vi "Puff_release3_chs.vi"() -> (5 "Plug in titles":string[](array[string]), 7 "Plug in values":string[](array[string]))   [LabVIEW 2011]
uses:
  Controls/Post_Process.ctl
  Globals/Plug_in_data_global.vi
  Globals/Meas_global.vi
  Globals/Constants_global.vi
  Globals/Dynamic_call_global.ph.vi
  <vilib>/Analysis/NI_AALPro.lvlib
panel:
  out "FFID Trace Variance":cluster{dbl, dbl, dbl[]}(graph)
  in  "Per Block Mode":T1(ring)
  in  "Averaging Samples":i32=1 min=1
  out "Valve to monitor delay (s)":dbl format="%.2f"
  out "Monitor trigger Index":dbl format="%.2f"
  out "Valve Trigger Index":dbl format="%.2f"
  out "Monitor FID":cluster{dbl, dbl, dbl[]}(graph)
  out "delay":dbl format="%.2f"
  out "Pulse Width":dbl format="%.2f"
  out "falltime":dbl format="%.2f"
  out "top":dbl format="%.2f"
  out "risetime":dbl format="%.2f"
  in  "Save Time pdf?":bool
  out "Pdf":cluster{"Axis":dbl[], dbl[]}(graph)
  in  "Histogram Time":dbl format="%.2f"
  out "Current Block No":i32
  in  "Save averaged traces?":bool
  in  "Pause Mode":T2(ring)
  in  "OK":bool
  out "No of Valid Blocks":dbl
  out "Valve Trace":dbl[](graph)
  out "FFID Trace":cluster{dbl, dbl, dbl[]}(graph)
  out "Source On":i32
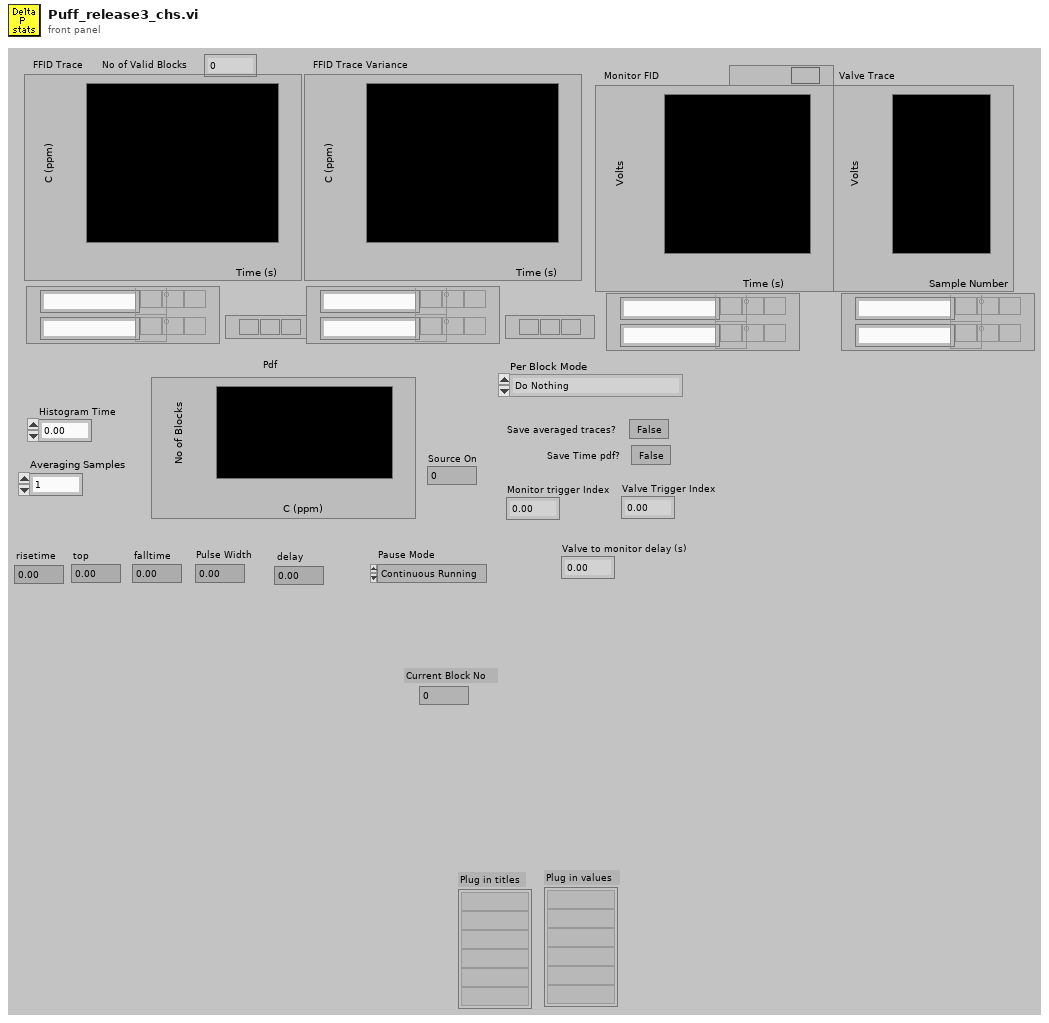
[diagram p1: front panel]
types:
  T1 = enum16{"Do Nothing", "Save Block Time Traces", "Save Jpeg plots"}
  T2 = enum16{"Continuous Running", "After Each  Block"}
  T3 = typedef "Post_Process.ctl" = enum16{"Take New Data", "Post Process Raw Data File"}
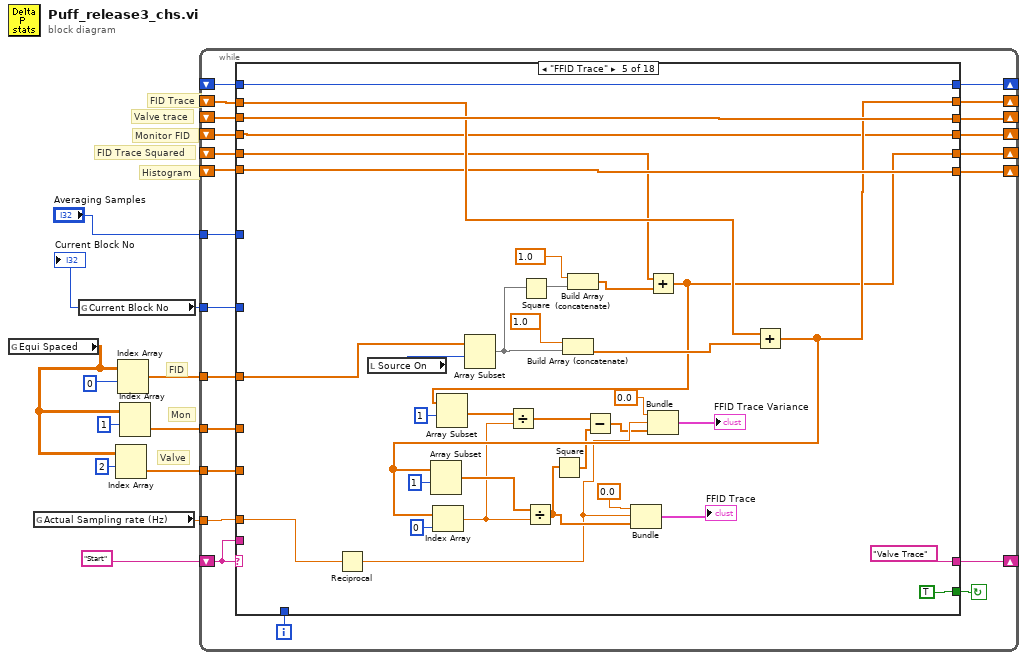
[diagram p0: block diagram]
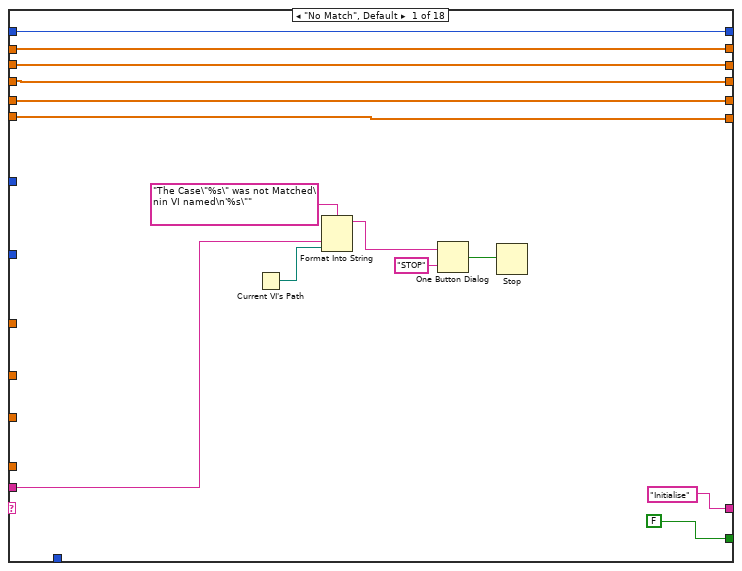
[diagram p2: hidden frame]
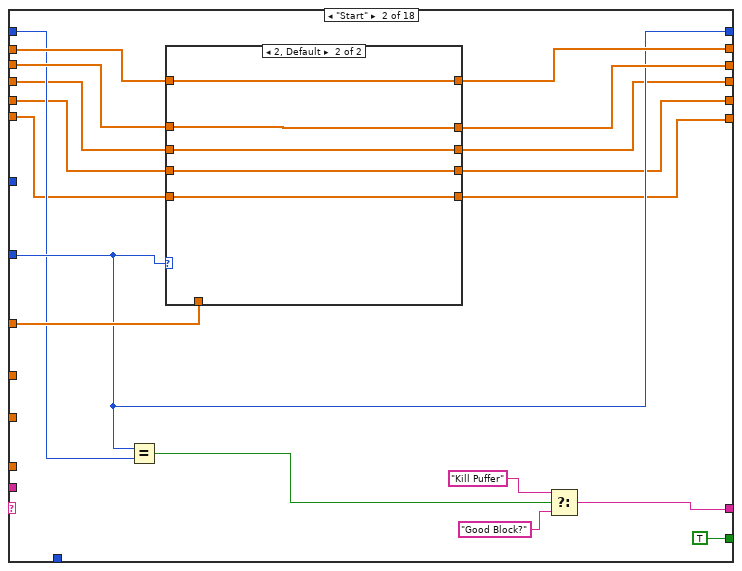
[diagram p3: hidden frame]
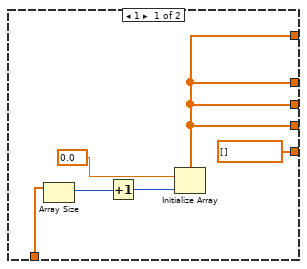
[diagram p4: hidden frame]
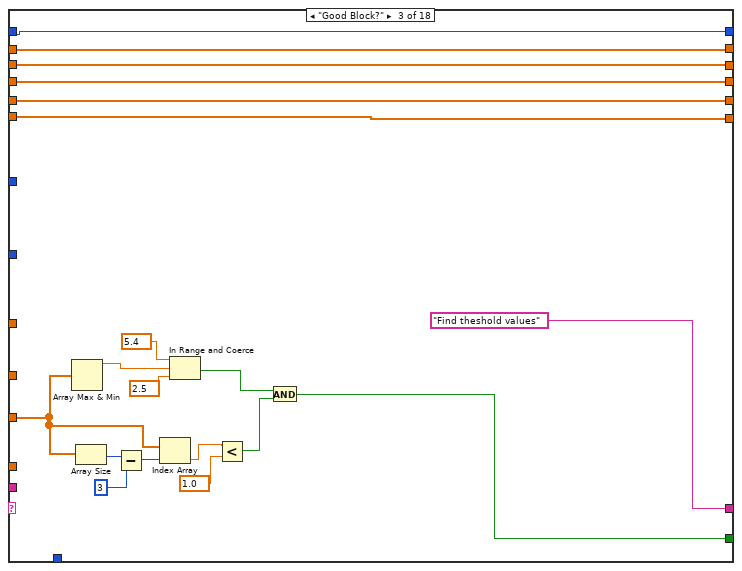
[diagram p5: hidden frame]
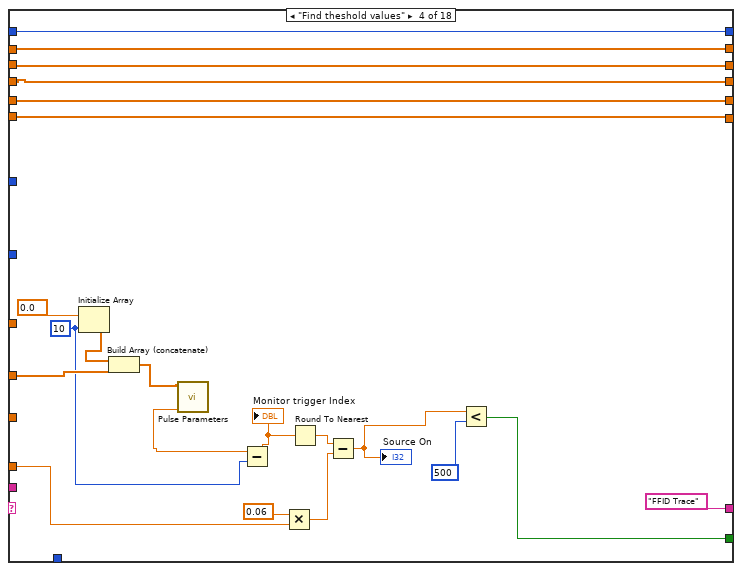
[diagram p6: hidden frame]
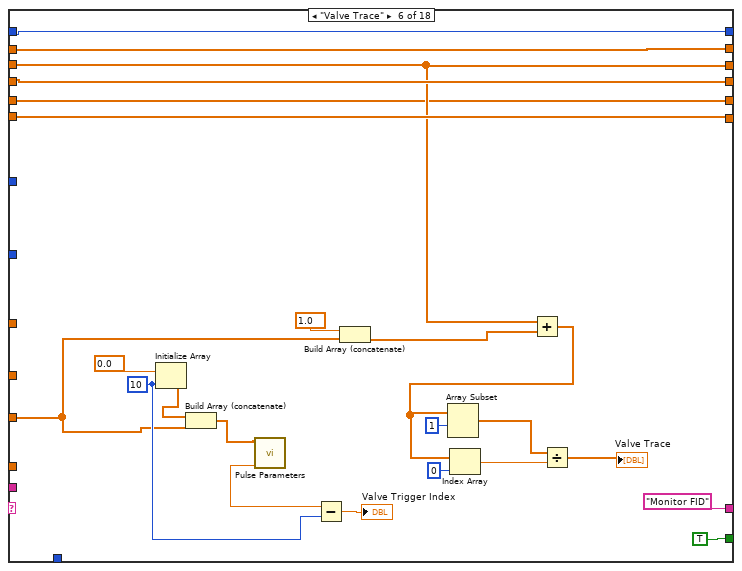
[diagram p7: hidden frame]
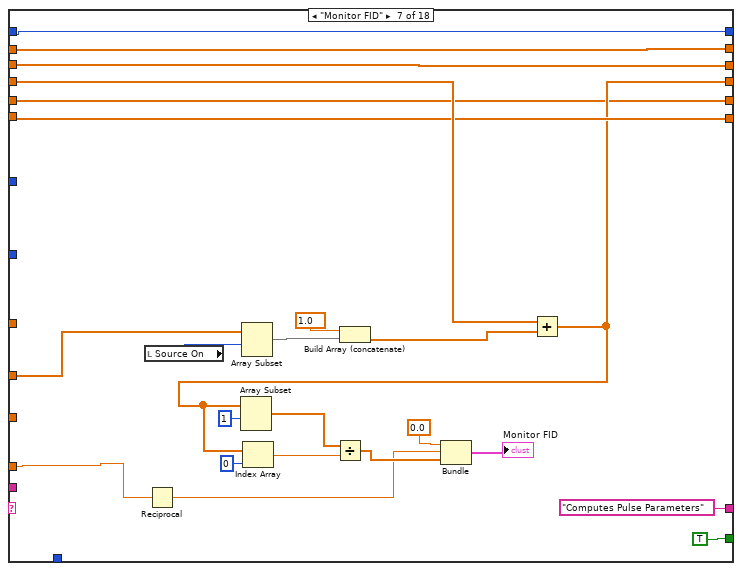
[diagram p8: hidden frame]
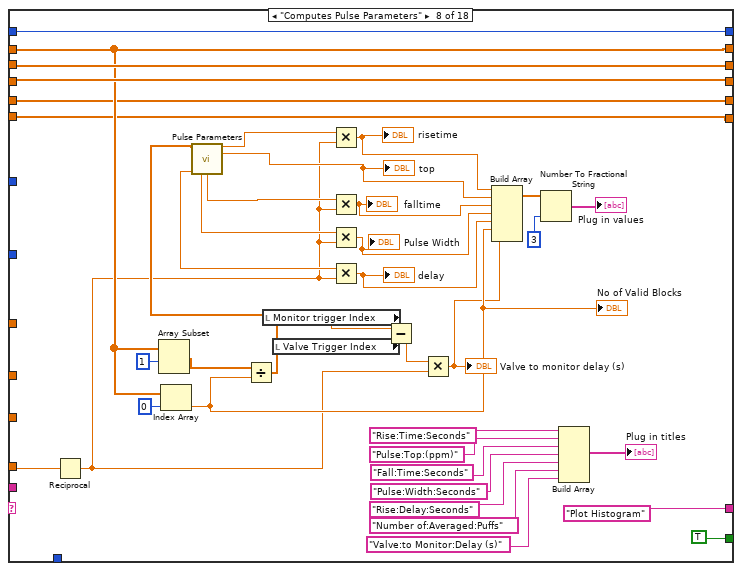
[diagram p9: hidden frame]
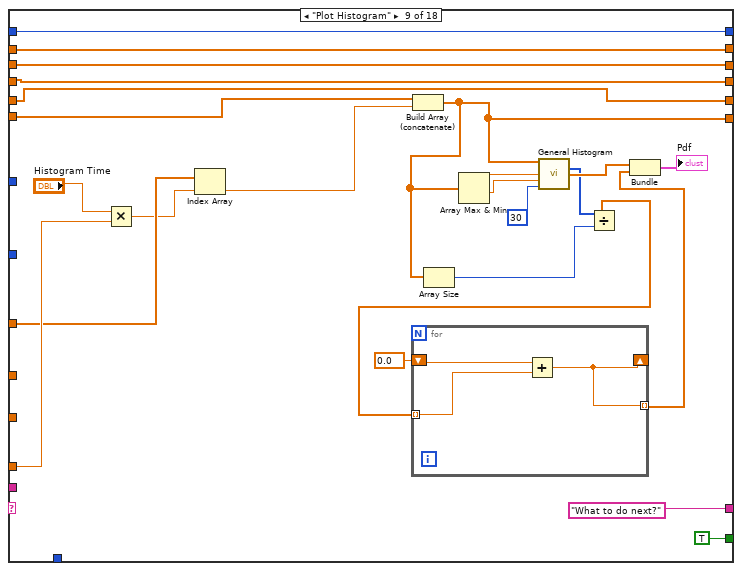
[diagram p10: hidden frame]
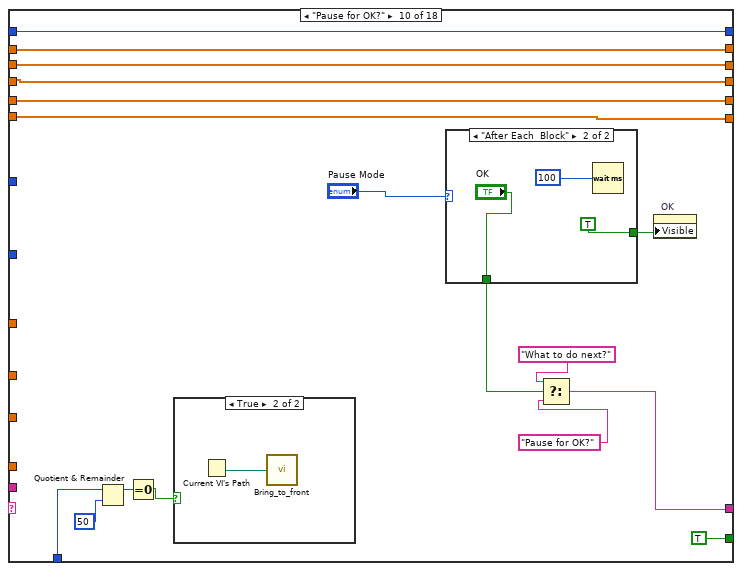
[diagram p11: hidden frame]
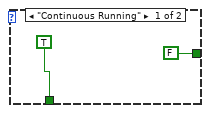
[diagram p13: hidden frame]
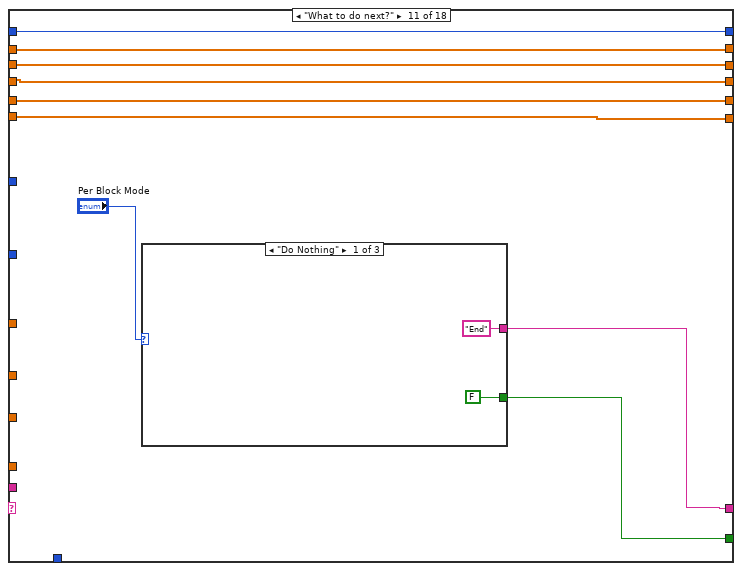
[diagram p14: hidden frame]
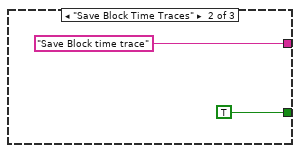
[diagram p15: hidden frame]
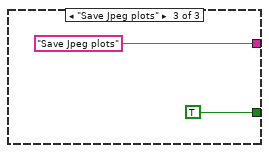
[diagram p16: hidden frame]
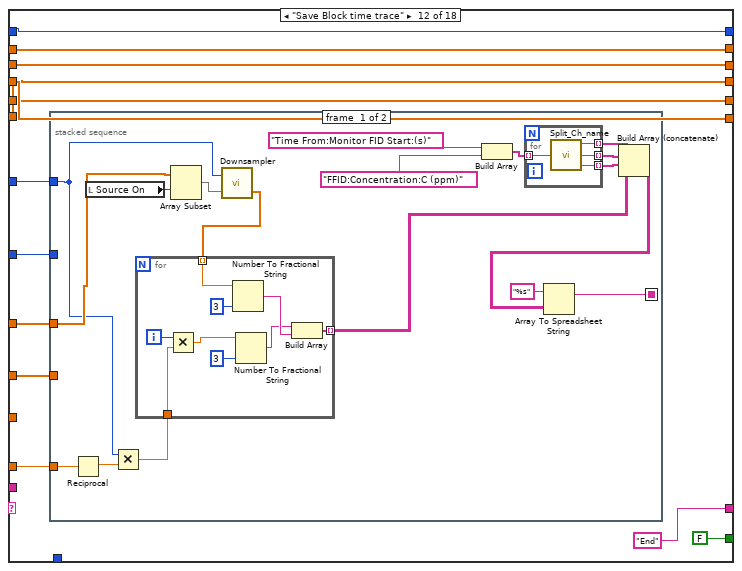
[diagram p17: hidden frame]
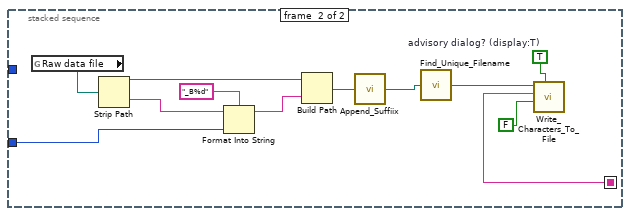
[diagram p18: hidden frame]
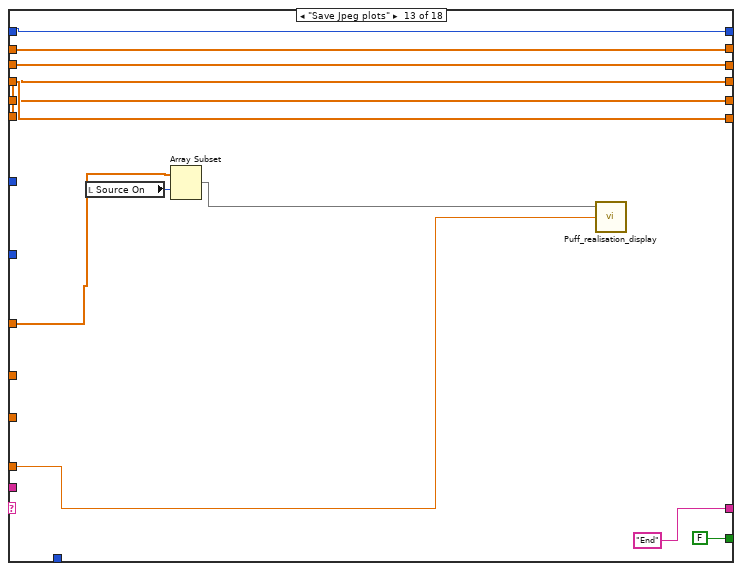
[diagram p19: hidden frame]
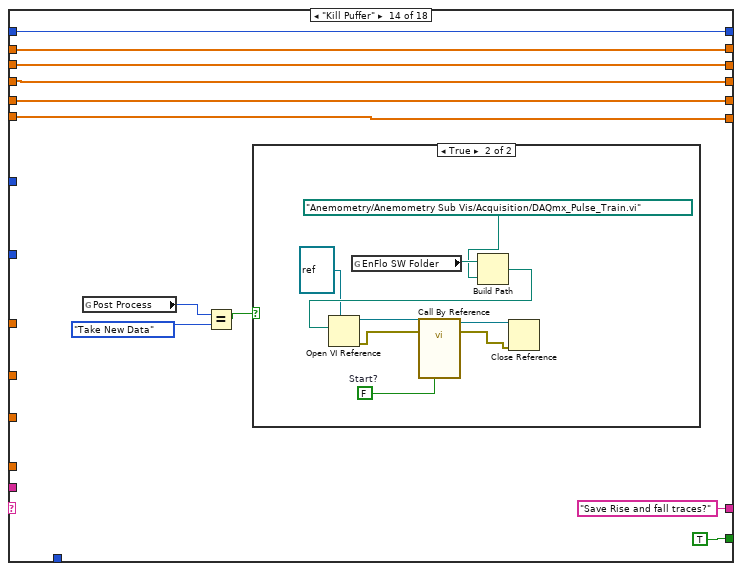
[diagram p20: hidden frame]
diagram:
  # "FID Trace Squared"
  # "Valve"
  # "Mon"
  # "FID"
  # "Histogram"
  # "Monitor FID"
  # "Valve trace"
  # "FID Trace"
  n1 = global read "Plug_in_data_global.vi" "Equi Spaced"() -> (w4:dbl[][])
  n2 = global read "Meas_global.vi" "Actual Sampling rate (Hz)"() -> (w8:dbl)
  n3 = global read "Meas_global.vi" "Current Block No"() -> (w7:i32)
  "Current Block No" <- w7
  n4 = Index Array(array=w4, index (row)=2) -> (element=w3:dbl[])  [unwired: 1 in]
  n5 = Index Array(array=w4, index (row)=0) -> (element=w9:dbl[])  [unwired: 1 in]
  n6 = Index Array(array=w4, index (row)=1) -> (element=w10:dbl[])  [unwired: 1 in]
  n7 = while {
    shift-left: "Start" -> [w31]
    shift-right: [w32] -> _
    shift-right: [w30] -> _
    shift-left: _ -> [w27]
    shift-right: [w29] -> _
    shift-left: _ -> [w28]
    tunnel: w10 -> [w26]
    tunnel: w9 -> [w25]
    tunnel: w8 -> [w24]
    tunnel: w7 -> [w23]
    shift-right: [w20] -> _
    shift-left: _ -> [w21]
    shift-right: [w18] -> _
    shift-left: _ -> [w19]
    shift-right: [w16] -> _
    shift-left: _ -> [w15]
    tunnel: w3 -> [w17]
    tunnel: "Averaging Samples" -> [w14]
    shift-right: [w12] -> _
    shift-left: _ -> [w13]
    i -> [w22]
    stop <- w33 continue-if-true
    n8 = case shown="\"FFID Trace\"" w31 {
      tunnel: [FALSE TRUE ("Processing last block?") w85 w112 TRUE ("Processing last block?") TRUE ("Processing last block?") TRUE ("Processing last block?") TRUE ("Processing last block?") TRUE ("Processing last block?") TRUE ("Processing last block?") w287 FALSE ("Processing last block?") FALSE ("Processing last block?") TRUE ("Processing last block?") w390 TRUE ("Processing last block?") "Save Time pdf?" FALSE ("Processing last block?")] -> w33
      tunnel: ["Initialise" w55 "Find theshold values" "FFID Trace" "Valve Trace" "Monitor FID" "Computes Pulse Parameters" "Plot Histogram" ("f") "What to do next?" ("f") w266 w288 "End" "End" "Save Rise and fall traces?" w393 "Save Time pdf?" "Save Time pdf" "End"] -> w32
      tunnel: w31 -> [w42 _ _ _ _ _ _ _ _ _ _ _ _ _ _ _ _ _]
      tunnel: [w39 w64 w95 w115 w137 w170 w191 w205 w259 w279 w294 w313 w368 w379 w399 w407 w477 w488] -> w30
      tunnel: [w38 w62 w94 w114 w148 w152 w188 w233 w258 w278 w293 w312 w367 w378 w398 w406 w476 w487] -> w29
      tunnel: w28 -> [w38 w61 w94 w114 w148 w152 w188 w233 w258 w278 w293 w312 w367 w378 w398 w406 w476 w487]
      tunnel: w27 -> [w39 w63 w95 w115 w146 w170 w191 w205 w259 w279 w294 w313 w368 w379 w399 w407 w477 w488]
      tunnel: w26 -> [_ _ _ w108 _ _ w175 _ _ _ _ w309 _ _ _ _ _ w484]
      tunnel: w25 -> [_ w60 _ _ w147 _ _ _ w254 _ _ w308 w361 _ _ _ _ w483]
      tunnel: w24 -> [_ _ _ w102 w135 _ w176 w231 w255 _ _ w302 w358 _ _ _ _ _]
      tunnel: w23 -> [_ w59 _ _ _ _ _ _ _ _ _ w307 _ _ _ _ _ w482]
      tunnel: w22 -> [_ _ _ _ _ _ _ _ _ w276 _ _ _ _ _ _ _ _]
      tunnel: w21 -> [w37 w58 w86 w111 w142 w169 w190 w229 w257 w272 w292 w306 w364 w375 _ w403 _ w481]
      tunnel: [w37 w59 w86 w111 w142 w169 w190 w229 w257 w272 w292 w306 w364 w375 0 w403 0 w481] -> w20
      tunnel: w19 -> [w36 w52 w84 w104 w141 w162 w186 w204 w251 w271 w291 w305 w363 w371 w391 w402 w472 w479]
      tunnel: [w36 w53 w84 w104 w141 w162 w186 w204 w243 w271 w291 w305 w363 w371 w391 w402 w472 w479] -> w18
      tunnel: w17 -> [_ _ w80 _ _ w155 _ _ _ _ _ _ _ _ _ _ _ _]
      tunnel: [w35 w51 w81 w105 w133 w163 w177 w209 w240 w270 w290 w304 w362 w370 w392 w401 w471 w480] -> w16
      tunnel: w15 -> [w35 w50 w81 w105 w133 w163 w187 w209 w240 w270 w290 w304 w362 w370 w392 w401 w471 w480]
      tunnel: w14 -> [_ _ _ _ _ _ _ _ _ _ _ w303 _ _ _ _ _ _]
      tunnel: w13 -> [w34 w48 w77 w96 w128 w151 w174 w197 w236 w263 w286 w301 w357 w369 w389 w400 w470 w478]
      tunnel: [w34 w49 w77 w96 w126 w151 w174 w197 w236 w263 w286 w301 w357 w369 w389 w400 w470 w478] -> w12
      frame "No Match", Default {
        n9 = Current VI's Path() -> (path=w41:path)
        n10 = Format Into String(format string="The Case\"%s\" was not Matched\nin VI named\n'%s\"" ("Format String"), w42, w41) -> (resulting string=w45:string)  [unwired: 2 in, 1 out]
        n11 = One Button Dialog(message=w45, button name ("OK")="STOP") -> (true=w43:bool)
        n12 = Stop(stop? (T)=w43) -> ()
      }
      frame "Start" {
        n13 = Equal?(x=w59, y=w58) -> (x = y?=w57:bool)
        n14 = case shown="2, Default" w59 {
          tunnel: [w66 w76] -> w64
          tunnel: w63 -> [_ w76]
          tunnel: [w66 w75] -> w62
          tunnel: w61 -> [_ w75]
          tunnel: w60 -> [w71 _]
          tunnel: [dbl[] [] w74] -> w53
          tunnel: w52 -> [_ w74]
          tunnel: [w66 w73] -> w51
          tunnel: w50 -> [_ w73]
          tunnel: [w66 w72] -> w49
          tunnel: w48 -> [_ w72]
          frame 1 {
            n15 = Array Size(array=w71) -> (size(s)=w70:i32)
            n16 = Increment(x=w70) -> (x+1=w67:i32)
            n17 = Initialize Array(0.0 ("element"), w67) -> (w66:dbl[])
          }
          frame 2, Default {
          }
        }
        n18 = Select(t="Kill Puffer", s=w57, f="Good Block?") -> (s? t:f=w55:string)
      }
      frame "Good Block?" {
        n19 = Array Max & Min(array=w80) -> (max value=w83:dbl)  [unwired: 3 out]
        n20 = Array Size(array=w80) -> (size(s)=w79:i32)
        n21 = Subtract(x=w79, y=3) -> (x-y=w91:i32)
        n22 = Index Array(array=w80, index=w91) -> (element=w90:dbl)
        n23 = In Range and Coerce(upper limit=5.4, x=w83, lower limit=2.5 ("y")) -> (In Range?=w87:bool)  [unwired: 1 out]
        n24 = Less?(x=w90, y=1.0) -> (x < y?=w88:bool)
        n25 = And(x=w87, y=w88) -> (x .and. y?=w85:bool)
      }
      frame "Find theshold values" {
        w106 = 10 ("dimension size")
        n26 = Initialize Array(0.0, w106) -> (w107:dbl[])
        n27 = Build Array (concatenate)(w107, w108) -> (w109:dbl[])
        n28 = call <vilib>:"Pulse Parameters.vi"("X"=w109) -> ("delay"=w101:dbl)  [unwired: 14 out]
        n29 = Subtract(x=w101, y=w106) -> (x-y=w100:dbl)
        "Monitor trigger Index" <- w100
        n30 = Multiply(x=0.06 ("y"), y=w102) -> (x*y=w98:dbl)
        n31 = Round To Nearest(number=w100) -> (nearest integer value=w99:dbl)
        n32 = Subtract(x=w99, y=w98) -> (x-y=w97:dbl)
        "Source On" <- w97
        n33 = Less?(x=w97, y=500) -> (x < y?=w112:bool)
      }
      frame "FFID Trace" {
        n34 = Reciprocal(x=w135) -> (1/x=w119:dbl)
        n35 = local read "Source On"() -> (w143:i32)
        n36 = Array Subset(array=w147, index=w143) -> (w131:dbl[])  [unwired: 1 in]
        n37 = Square(x=w131) -> (x^2=w130:dbl[])
        n38 = Build Array (concatenate)(1.0, w131) -> (w144:dbl[])
        n39 = Build Array (concatenate)(1.0, w130) -> (w129:dbl[])
        n40 = Add(x=w128, y=w129) -> (x+y=w126:dbl[])
        n41 = Array Subset(array=w126, index=1) -> (w125:dbl[])  [unwired: 1 in]
        n42 = Add(x=w146, y=w144) -> (x+y=w137:dbl[])
        n43 = Array Subset(array=w137, index=1) -> (w136:dbl[])  [unwired: 1 in]
        n44 = Index Array(array=w137, index=0) -> (element=w124:dbl)
        n45 = Divide(x=w125, y=w124) -> (x/y=w122:dbl[])
        n46 = Divide(x=w136, y=w124) -> (x/y=w123:dbl[])
        n47 = Square(x=w123) -> (x^2=w121:dbl[])
        n48 = Subtract(x=w122, y=w121) -> (x-y=w118:dbl[])
        n49 = Bundle(0.0, w119, w123) -> (→"FFID Trace":cluster{dbl, dbl, dbl[]})  [unwired: 1 out]
        n50 = Bundle(0.0, w119, w118) -> (→"FFID Trace Variance":cluster{dbl, dbl, dbl[]})  [unwired: 1 out]
      }
      frame "Valve Trace" {
        w156 = 10 ("dimension size")
        n51 = Initialize Array(0.0, w156) -> (w157:dbl[])
        n52 = Build Array (concatenate)(w157, w155) -> (w158:dbl[])
        n53 = call <vilib>:"Pulse Parameters.vi"("X"=w158) -> ("delay"=w153:dbl)  [unwired: 14 out]
        n54 = Subtract(x=w153, y=w156) -> (x-y=→"Valve Trigger Index":dbl)
        n55 = Build Array (concatenate)(1.0, w155) -> (w171:dbl[])
        n56 = Add(x=w152, y=w171) -> (x+y=w160:dbl[])
        n57 = Array Subset(array=w160, index=1) -> (w165:dbl[])  [unwired: 1 in]
        n58 = Index Array(array=w160, index=0) -> (element=w164:dbl)
        n59 = Divide(x=w165, y=w164) -> (x/y=→"Valve Trace":dbl[])
      }
      frame "Monitor FID" {
        n60 = local read "Source On"() -> (w193:i32)
        n61 = Reciprocal(x=w176) -> (1/x=w179:dbl)
        n62 = Array Subset(array=w175, index=w193) -> (w192:dbl[])  [unwired: 1 in]
        n63 = Build Array (concatenate)(1.0, w192) -> (w194:dbl[])
        n64 = Add(x=w187, y=w194) -> (x+y=w177:dbl[])
        n65 = Array Subset(array=w177, index=1) -> (w181:dbl[])  [unwired: 1 in]
        n66 = Index Array(array=w177, index=0) -> (element=w180:dbl)
        n67 = Divide(x=w181, y=w180) -> (x/y=w185:dbl[])
        n68 = Bundle(0.0, w179, w185) -> (→"Monitor FID":cluster{dbl, dbl, dbl[]})  [unwired: 1 out]
      }
      frame "Computes Pulse Parameters" {
        n69 = Reciprocal(x=w231) -> (1/x=w200:dbl)
        n70 = Array Subset(array=w205, index=1) -> (w208:dbl[])  [unwired: 1 in]
        n71 = Index Array(array=w205, index=0) -> (element=w207:dbl)
        "No of Valid Blocks" <- w207
        n72 = Divide(x=w208, y=w207) -> (x/y=w206:dbl[])
        n73 = call <vilib>:"Pulse Parameters.vi"("X"=w206) -> ("risetime"=w228:dbl, "top"=w214:dbl, "delay"=w225:dbl, "duration"=w226:dbl, "falltime"=w227:dbl)  [unwired: 10 out]
        "top" <- w214
        n74 = local read "Monitor trigger Index"() -> (w202:dbl)
        n75 = local read "Valve Trigger Index"() -> (w203:dbl)
        n76 = Multiply(x=w228, y=w200) -> (x*y=w213:dbl)
        "risetime" <- w213
        n77 = Multiply(x=w227, y=w200) -> (x*y=w212:dbl)
        "falltime" <- w212
        n78 = Multiply(x=w226, y=w200) -> (x*y=w211:dbl)
        "Pulse Width" <- w211
        n79 = Multiply(x=w225, y=w200) -> (x*y=w210:dbl)
        "delay" <- w210
        n80 = Subtract(x=w202, y=w203) -> (x-y=w201:dbl)
        n81 = Multiply(x=w201, y=w200) -> (x*y=w199:dbl)
        "Valve to monitor delay (s)" <- w199
        n82 = Build Array(w213, w214, w212, w211, w210, w207, w199) -> (w224:dbl[])
        n83 = Number To Fractional String(number=w224, precision (6)=i16 3) -> (F-format string=→"Plug in values":string[])  [unwired: 2 out]
        n84 = Build Array("Rise:Time:Seconds", "Pulse:Top:(ppm)", "Fall:Time:Seconds", "Pulse:Width:Seconds", "Rise:Delay:Seconds", "Number of:Averaged:Puffs", "Valve:to Monitor:Delay (s)") -> (→"Plug in titles":string[])
      }
      frame "Plot Histogram" {
        n85 = Multiply(x="Histogram Time", y=w255) -> (x*y=w253:dbl)
        n86 = Index Array(array=w254, index=w253) -> (element=w252:dbl)
        n87 = Build Array (concatenate)(w251, w252) -> (w243:dbl[])
        n88 = Array Size(array=w243) -> (size(s)=w241:i32)
        n89 = Array Max & Min(array=w243) -> (max value=w250:dbl, min value=w249:dbl)  [unwired: 2 out]
        n90 = call <vilib>:"General Histogram.vi"("X"=w243, "max"=w250, "min"=w249, "# bins"=30) -> ("Histogram"=w242:i32[], "Axis"=w247:dbl[])  [unwired: 2 in, 8 out]
        n91 = Divide(x=w242, y=w241) -> (x/y=w237:dbl[])
        n92 = for {
          shift-right: [w260] -> _
          shift-left: 0.0 -> [w262]
          tunnel: w237 -> [w261] mode=indexing
          tunnel: [w260] -> w238 mode=indexing
          n93 = Add(x=w262, y=w261) -> (x+y=w260:dbl)
        }
        n94 = Bundle("Axis"=w247, w238) -> (→"Pdf":cluster{"Axis":dbl[], dbl[]})  [unwired: 1 out]
      }
      frame "Pause for OK?" {
        n95 = Quotient & Remainder(x=w276, y=50) -> (x-y*floor(x/y)=w274:i32)  [unwired: 1 out]
        n96 = Equal To 0?(x=w274) -> (x = 0?=w273:bool)
        n97 = case shown="True" w273 {
          frame False {
          }
          frame True {
            n98 = Current VI's Path() -> (path=w280:path)
            n99 = call "Bring_to_front.vi"("path"=w280) -> ()
          }
        }
        n100 = case shown="\"After Each  Block\"" "Pause Mode" {
          tunnel: [TRUE "OK"] -> w267
          tunnel: [FALSE TRUE] -> w277
          frame "Continuous Running" {
          }
          frame "After Each  Block" {
            n101 = Wait (ms)(milliseconds to wait=u32 100 ("f")) -> ()  [unwired: 1 out]
          }
        }
        n102 = Select(t="What to do next?" ("f"), s=w267, f="Pause for OK?") -> (s? t:f=w266:string)
        n103 = property on="OK" class="Bool"("Visible"=w277) -> ()  [unwired: 2 in, 2 out]
      }
      frame "What to do next?" {
        n104 = case shown="\"Do Nothing\"" "Per Block Mode" {
          tunnel: ["End" ("t") "Save Block time trace" ("t") "Save Jpeg plots" ("t")] -> w288
          tunnel: [FALSE TRUE TRUE] -> w287
          frame "Do Nothing" {
          }
          frame "Save Block Time Traces" {
          }
          frame "Save Jpeg plots" {
          }
        }
      }
      frame "Save Block time trace" {
        n105 = stacked-sequence {
          seq-local: [w327 _] -> [_ w353]
          tunnel: w309 -> [_ _]
          tunnel: w308 -> [w324 _]
          tunnel: w307 -> [_ w350]
          tunnel: w303 -> [w319 _]
          tunnel: w302 -> [w321 _]
          frame #0 {
            n106 = Reciprocal(x=w321) -> (1/x=w320:dbl)
            n107 = local read "Source On"() -> (w325:i32)
            n108 = Multiply(x=w319, y=w320) -> (x*y=w318:dbl)
            n109 = Array Subset(array=w324, index=w325) -> (w323:dbl[])  [unwired: 1 in]
            n110 = call "Downsampler.vi"("Input Array"=w323, "Averaging samples"=w319) -> ("Downsampled Array"=w322:dbl[])  [unwired: 1 out]
            n111 = for {
              tunnel: [w342] -> w326 mode=indexing
              tunnel: w322 -> [w339] mode=indexing
              tunnel: w318 -> [w338]
              i -> [w337]
              n112 = Multiply(x=w337, y=w338) -> (x*y=w336:dbl)
              n113 = Number To Fractional String(number=w339, precision (6)=i16 3) -> (F-format string=w341:string)  [unwired: 2 out]
              n114 = Number To Fractional String(number=w336, precision (6)=i16 3) -> (F-format string=w340:string)  [unwired: 2 out]
              n115 = Build Array(w340, w341) -> (w342:string[])
            }
            n116 = Build Array("Time From:Monitor FID Start:(s)", "FFID:Concentration:C (ppm)") -> (w317:string[])
            n117 = for {
              tunnel: w317 -> [w335] mode=indexing
              tunnel: [w334] -> w316 mode=indexing
              tunnel: [w333] -> w315 mode=indexing
              tunnel: [w332] -> w314 mode=indexing
              n118 = call "Split_Ch_name.vi"("Ch name"=w335) -> ("Top level"=w334:string, "Middle"=w333:string, "Low level"=w332:string)
            }
            n119 = Build Array (concatenate)(w316, w315, w314, w326) -> (w329:string[][])
            n120 = Array To Spreadsheet String(array=w329, 3:"%s" ("format string")) -> (spreadsheet string=w327:string)  [unwired: 1 out]
          }
          frame #1 {
            w355 = TRUE  # advisory dialog? (display:T)
            n121 = global read "Meas_global.vi" "Raw data file"() -> (w356:path)
            n122 = Strip Path(path=w356) -> (stripped path=w352:path, name=w351:string)
            n123 = Format Into String(format string="_B%d", initial string=w351, w350) -> (resulting string=w348:string)  [unwired: 1 in, 1 out]
            n124 = Build Path(base path=w352, name or relative path=w348) -> (appended path=w347:path)
            n125 = call "Append_Suffiix.vi"("Results file"=w347) -> ("appended path"=w346:path)
            n126 = call "Find_Unique_Filename.vi"("Path In"=w346) -> ("Unique Path Out"=w345:path)  [unwired: 1 in, 1 out]
            n127 = call "Write_Characters_To_File.vi"("file path (dialog if empty)"=w345, "advisory dialog? (display:T)"=w355, "character string"=w353, "append to file? (new file:F)"=FALSE) -> ()  [unwired: 1 in, 4 out]
          }
        }
      }
      frame "Save Jpeg plots" {
        n128 = local read "Source On"() -> (w360:i32)
        n129 = Array Subset(array=w361, index=w360) -> (w359:dbl[])  [unwired: 1 in]
        n130 = call "Puff_realisation_display.vi"("Actual Sampling rate (Hz)"=w358, "Input Array"=w359) -> ()  [unwired: 2 out]
      }
      frame "Kill Puffer" {
        n131 = global read "Meas_global.vi" "Post Process"() -> (w374:T3)
        n132 = Equal?(x=w374, y=Post_Process."Take New Data" ("Post Process")) -> (x = y?=w372:bool)
        n133 = case shown="True" w372 {
          frame False {
          }
          frame True {
            w388 = FALSE  # Start?
            n134 = global read "Constants_global.vi" "EnFlo SW Folder"() -> (w387:path)
            n135 = Build Path(base path=w387, name or relative path=path "Anemometry/Anemometry Sub Vis/Acquisition/DAQmx_Pulse_Train.vi") -> (appended path=w385:path)
            n136 = Open VI Reference(type specifier VI Refnum (for type only)=refnum<vi> refnum, vi path=w385) -> (vi reference=w384:refnum<vi>, error out=w381:errorcluster)  [unwired: 1 in, 3 out]
            n137 = call-by-ref "?"(reference=w384, error in=w381, "Start?"=w388) -> (reference out=w382:refnum<vi>, error out=w380:errorcluster)  [unwired: 8 in]
            n138 = Close Reference(reference=w382, error in (no error)=w380) -> ()  [unwired: 1 out]
          }
        }
      }
      frame "Save Rise and fall traces?" {
        n139 = Select(t="Write Results file", s="Save averaged traces?", f="Save Time PDF?") -> (s? t:f=w393:string)
        n140 = global read "Meas_global.vi" "Processing last block?"() -> (w390:bool)
      }
      frame "Write Results file" {
        n141 = stacked-sequence {
          seq-local: [w416 _] -> [_ w446]
          frame #0 {
            n142 = local read "FFID Trace"() -> (w426:cluster{dbl, dbl, dbl[]})
            n143 = local read "Monitor FID"() -> (w415:cluster{dbl, dbl, dbl[]})
            n144 = Unbundle(w426) -> (w424:dbl, w425:dbl, w423:dbl[])
            n145 = Unbundle(w415) -> (w414:dbl[])  [unwired: 2 out]
            n146 = for {
              tunnel: w425 -> [w437]
              tunnel: w424 -> [w436]
              tunnel: w423 -> [w431] mode=indexing
              tunnel: [w434] -> w421 mode=indexing
              tunnel: w414 -> [w432] mode=indexing
              i -> [w438]
              n147 = Multiply(x=w437, y=w438) -> (x*y=w435:dbl)
              n148 = Add(x=w436, y=w435) -> (x+y=w433:dbl)
              n149 = Build Array(w433, w432, w431) -> (w434:dbl[])
            }
            n150 = Build Array("Time From:Monitor FID Start:(s)", "Monitor FID:Voltage:Trace", "FFID:Concentration:C (ppm)") -> (w411:string[])
            n151 = for {
              tunnel: w411 -> [w430] mode=indexing
              tunnel: [w429] -> w410 mode=indexing
              tunnel: [w428] -> w409 mode=indexing
              tunnel: [w427] -> w408 mode=indexing
              n152 = call "Split_Ch_name.vi"("Ch name"=w430) -> ("Top level"=w429:string, "Middle"=w428:string, "Low level"=w427:string)
            }
            n153 = Number To Fractional String(number=w421, precision (6)=i16 3) -> (F-format string=w420:string[][])  [unwired: 2 out]
            n154 = Build Array (concatenate)(w410, w409, w408, w420) -> (w418:string[][])
            n155 = Array To Spreadsheet String(array=w418, 3:"%s" ("format string")) -> (spreadsheet string=w416:string)  [unwired: 1 out]
          }
          frame #1 {
            w461 = TRUE  # advisory dialog? (display:T)
            n156 = global read "Dynamic_call_global.ph.vi" "Plug in titles"() -> (w458:string[])
            n157 = global read "Dynamic_call_global.ph.vi" "Plug in values"() -> (w454:string[])
            n158 = global read "Meas_global.vi" "Raw data file"() -> (w465:path)
            n159 = Strip Path(path=w465) -> (stripped path=w459:path, name=w444:string)
            n160 = String Subset(string=w444, offset (0)=0, length (rest)=28 ("length (rest)")) -> (substring=w441:string)
            n161 = for {
              tunnel: w458 -> [w469] mode=indexing
              tunnel: [w468] -> w457 mode=indexing
              tunnel: [w467] -> w456 mode=indexing
              tunnel: [w466] -> w455 mode=indexing
              n162 = call "Split_Ch_name.vi"("Ch name"=w469) -> ("Top level"=w468:string, "Middle"=w467:string, "Low level"=w466:string)
            }
            n163 = Concatenate Strings(w441, "_Av" ("string")) -> (w464:string)
            n164 = Initialize Array("", 15) -> (w451:string[])
            n165 = Build Path(base path=w459, name or relative path=w464) -> (appended path=w440:path)
            n166 = call "Append_Suffiix.vi"("Results file"=w440) -> ("appended path"=w439:path)
            n167 = call "Asterisk_header.vi"("Channel names"=w451) -> ("Header string"=w447:string)
            n168 = call "Find_Unique_Filename.vi"("Path In"=w439) -> ("Unique Path Out"=w462:path)  [unwired: 1 in, 1 out]
            n169 = Build Array(w457, w456, w455, w454) -> (w452:string[][])
            n170 = Array To Spreadsheet String(array=w452, 3:"%s" ("format string")) -> (spreadsheet string=w448:string)  [unwired: 1 out]
            n171 = Concatenate Strings(w448, w447, w446) -> (w445:string)
            n172 = call "Write_Characters_To_File.vi"("file path (dialog if empty)"=w462, "advisory dialog? (display:T)"=w461, "character string"=w445, "append to file? (new file:F)"=FALSE) -> ()  [unwired: 1 in, 4 out]
          }
        }
      }
      frame "Save Time pdf?" {
      }
      frame "Save Time pdf" {
        n173 = stacked-sequence {
          seq-local: [w497 _] -> [_ w518]
          tunnel: w484 -> [_ _]
          tunnel: w483 -> [_ _]
          tunnel: w482 -> [_ _]
          frame #0 {
            n174 = local read "Pdf"() -> (w495:cluster{"Axis":dbl[], dbl[]})
            n175 = Unbundle(w495) -> ("Axis"=w494:dbl[], w493:dbl[])
            n176 = for {
              tunnel: w493 -> [w511] mode=indexing
              tunnel: w494 -> [w510] mode=indexing
              tunnel: [w509] -> w496 mode=indexing
              n177 = Number To Fractional String(number=w511, precision (6)=i16 3) -> (F-format string=w507:string)  [unwired: 2 out]
              n178 = Number To Fractional String(number=w510, precision (6)=i16 3) -> (F-format string=w508:string)  [unwired: 2 out]
              n179 = Build Array(w508, w507) -> (w509:string[])
            }
            n180 = Build Array("FFID:Concentration:C (ppm)", "Pdf:Bin:Frequency") -> (w492:string[])
            n181 = for {
              tunnel: w492 -> [w505] mode=indexing
              tunnel: [w504] -> w491 mode=indexing
              tunnel: [w503] -> w490 mode=indexing
              tunnel: [w502] -> w489 mode=indexing
              n182 = call "Split_Ch_name.vi"("Ch name"=w505) -> ("Top level"=w504:string, "Middle"=w503:string, "Low level"=w502:string)
            }
            n183 = Build Array (concatenate)(w491, w490, w489, w496) -> (w499:string[][])
            n184 = Array To Spreadsheet String(array=w499, 3:"%s" ("format string")) -> (spreadsheet string=w497:string)  [unwired: 1 out]
          }
          frame #1 {
            w536 = TRUE  # advisory dialog? (display:T)
            n185 = global read "Dynamic_call_global.ph.vi" "Plug in titles"() -> (w530:string[])
            n186 = global read "Dynamic_call_global.ph.vi" "Plug in values"() -> (w526:string[])
            n187 = global read "Meas_global.vi" "Raw data file"() -> (w539:path)
            n188 = local read "Histogram Time"() -> (w531:dbl)
            n189 = Strip Path(path=w539) -> (stripped path=w534:path, name=w514:string)
            n190 = String Subset(string=w514, offset (0)=0, length (rest)=20 ("length (rest)")) -> (substring=w513:string)
            n191 = for {
              tunnel: w530 -> [w543] mode=indexing
              tunnel: [w542] -> w529 mode=indexing
              tunnel: [w541] -> w528 mode=indexing
              tunnel: [w540] -> w527 mode=indexing
              n192 = call "Split_Ch_name.vi"("Ch name"=w543) -> ("Top level"=w542:string, "Middle"=w541:string, "Low level"=w540:string)
            }
            n193 = Format Into String(format string="_T=%.2f", initial string=w513, w531) -> (resulting string=w532:string)  [unwired: 1 in, 1 out]
            n194 = Initialize Array("", 15) -> (w523:string[])
            n195 = Build Path(base path=w534, name or relative path=w532) -> (appended path=w538:path)
            n196 = call "Asterisk_header.vi"("Channel names"=w523) -> ("Header string"=w519:string)
            n197 = call "Find_Unique_Filename.vi"("Path In"=w538) -> ("Unique Path Out"=w537:path)  [unwired: 1 in, 1 out]
            n198 = Build Array(w529, w528, w527, w526) -> (w524:string[][])
            n199 = Array To Spreadsheet String(array=w524, 3:"%s" ("format string")) -> (spreadsheet string=w520:string)  [unwired: 1 out]
            n200 = Concatenate Strings(w520, w519, w518) -> (w517:string)
            n201 = call "Write_Characters_To_File.vi"("file path (dialog if empty)"=w537, "advisory dialog? (display:T)"=w536, "character string"=w517, "append to file? (new file:F)"=FALSE) -> ()  [unwired: 1 in, 4 out]
          }
        }
      }
    }
  }
